vi "20T_Set_Values.vi"   [LabVIEW 2016]
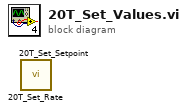
[diagram p0: block diagram]
diagram:
  n1 = call "20T_Set_Rate.vi"() -> ()  [unwired: 11 in, 1 out]
  n2 = call "20T_Set_Setpoint.vi"() -> ()  [unwired: 11 in, 1 out]
